vi "Drive Train Global.vi"() -> ()   [LabVIEW 2018]
panel:
  in  "Wheel Angle Offsets Practice Bot":T1={"FrontLeft"=-109.3, "FrontRight"=-174.2, "BackLeft"=-6.5, "BackRight"=140.0}
  in  "Angle Locking to":dbl=990.0
  in  "Angle to Lock To":dbl=270.0
  out "Lock to Angle":bool
  out "Robot Centric":bool
  in  "Don't Turn While Translate PID Gains":T2 {"derivative time (Td, min)" format="%.3f"; "integral time (Ti, min)" format="%.3f"; "proportional gain (Kc)" format="%.3f"}
  in  "Zero Yaw":bool
  in  "Wheel Angle Offsets":T1={"FrontLeft"=-37.4, "FrontRight"=-86.8, "BackLeft"=-65.8, "BackRight"=178.0}
  out "Wheel Angles":T1={"FrontLeft"=-0.07875069353355713, "FrontRight"=-0.07271635703058621, "BackLeft"=-0.09536056916057589, "BackRight"=-0.006532067663300722}
  in  "Rot. Point Y":dbl
  in  "Rot. Point X":dbl
  in  "Wheel Turn PID Values":T3={"Front Left"={"P Value"=0.014, "I Value"=0.0, "D Value"=0.0}, "Front Right"={"P Value"=0.014, "I Value"=0.0, "D Value"=0.0}, "Back Left"={"P Value"=0.014, "I Value"=0.0, "D Value"=0.0}, "Back Right"={"P Value"=0.014, "I Value"=0.0, "D Value"=0.0}}
  in  "Z Command":dbl=-0.0
  in  "Y Command":dbl
  out "Gyro Information":T4={"Rollover"=-1.0, "Yaw"=151.38, "Cont Yaw"=-208.62}
  in  "X Command":dbl=-0.0
  in  "Current State":enum16{"Reached Position", "Going to Position"}(ring)
  in  "Current Mode":T5(ring)=enum."Field Oriented"
  out "Extra Info":bool
  out "Velocity":cluster{"X":dbl, "Y":dbl, "Z":dbl}
  out "Position":cluster{"X":dbl, "Y":dbl, "Z":dbl}
  out "Wheel Drive Encoders":T6
  # "X Command is spin"
  # "Z is X"
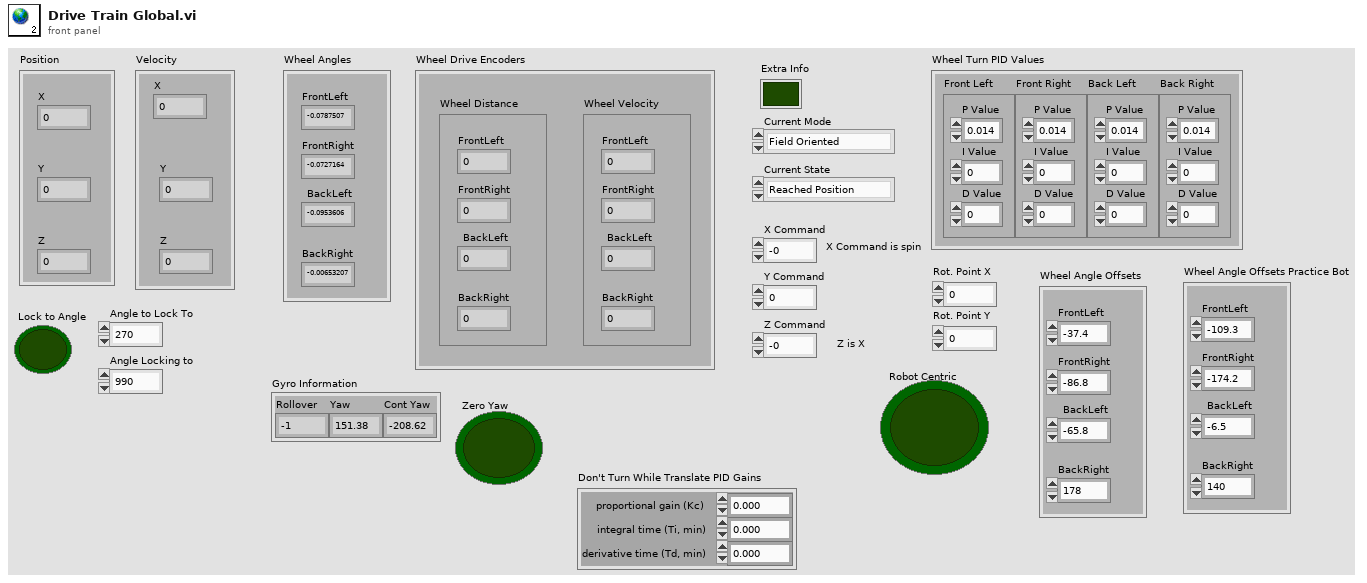
[diagram p1: front panel]
types:
  T1 = cluster{"FrontLeft":dbl, "FrontRight":dbl, "BackLeft":dbl, "BackRight":dbl}
  T2 = cluster{"proportional gain (Kc)":dbl, "integral time (Ti, min)":dbl, "derivative time (Td, min)":dbl}
  T3 = cluster{"Front Left":cluster{"P Value":dbl, "I Value":dbl, "D Value":dbl}, "Front Right":cluster{"P Value":dbl, "I Value":dbl, "D Value":dbl}, "Back Left":cluster{"P Value":dbl, "I Value":dbl, "D Value":dbl}, "Back Right":cluster{"P Value":dbl, "I Value":dbl, "D Value":dbl}}
  T4 = cluster{"Rollover":dbl, "Yaw":dbl, "Cont Yaw":dbl}
  T5 = enum16{"Autonomous Mode", "Field Oriented", "Robot Oriented", "Tank Mode"}
  T6 = cluster{"Wheel Velocity":cluster{"FrontLeft":dbl, "FrontRight":dbl, "BackLeft":dbl, "BackRight":dbl}, "Wheel Distance":cluster{"FrontLeft":dbl, "FrontRight":dbl, "BackLeft":dbl, "BackRight":dbl}}
diagram:
